vi "Updated_File_Copy.vi"(2 "Target Path":path, 3 "Source Path":path) -> (0 "error in (no error)":errorcluster)   [LabVIEW 2011]
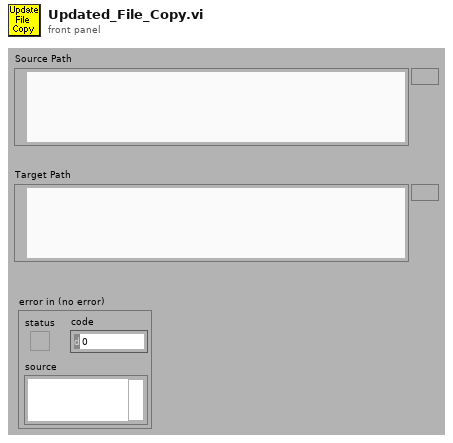
[diagram p1: front panel]
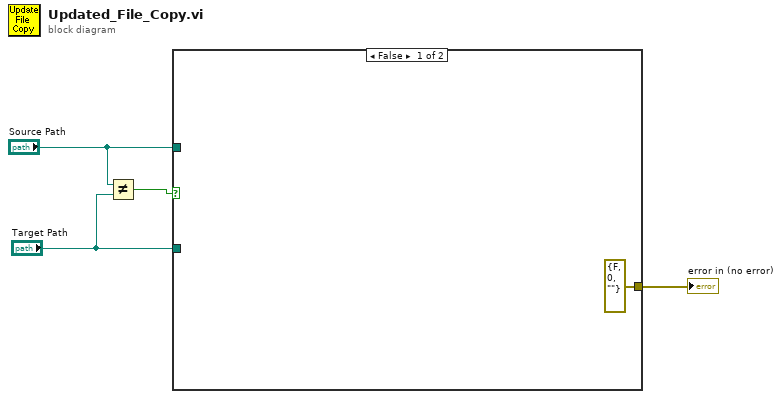
[diagram p0: block diagram]
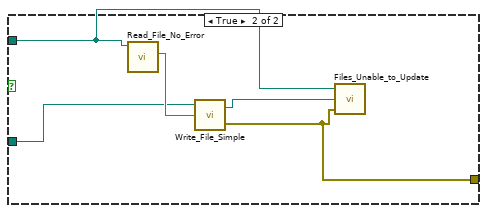
[diagram p2: hidden frame]
diagram:
  n1 = Not Equal?(x="Source Path", y="Target Path") -> (x != y?=w1:bool)
  n2 = case shown="False" w1 {
    tunnel: [errorcluster {"status"=FALSE, "code"=0, "source"=""} ("error out") w9] -> w4
    tunnel: "Target Path" -> [_ w7]
    tunnel: "Source Path" -> [_ w6]
    frame False {
    }
    frame True {
      n3 = call "Read_File_No_Error.vi"("Filename"=w6) -> ("string"=w10:string)  [unwired: 2 in, 7 out]
      n4 = call "Write_File_Simple.vi"("character string"=w10, "file path"=w7) -> ("error out"=w9:errorcluster, "file path Out"=w8:path)  [unwired: 1 in]
      n5 = call "Files_Unable_to_Update.vi"("error in (no error)"=w9, "Target Path"=w8, "Source Path"=w6) -> ()  [unwired: 1 out]
    }
  }
  "error in (no error)" <- w4
